vi "Parse.vi"(8 "error in (no error)":errorcluster, 11 "Multipart Parser in":refnum<class "Multipart Parser.lvclass">) -> (0 "error out":errorcluster, 1 "Stream":refnum<k5>, 3 "Request":refnum<class "Request.lvclass">)   [LabVIEW 2020, in "HTTP Utils.lvlib" / "Multipart Parser.lvclass"]
uses:
  Multipart Parser.lvclass
  Request/Request.lvclass
  Multipart Parser.lvclass/Multipart Parser.ctl
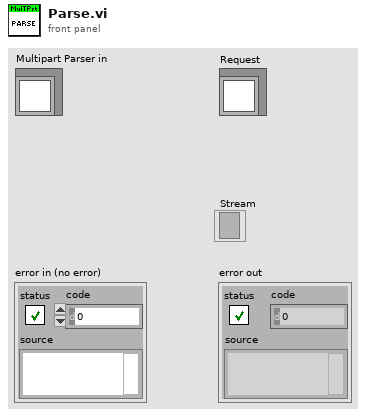
[diagram p1: front panel]
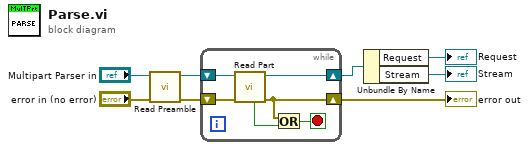
[diagram p0: block diagram]
diagram:
  n1 = call "Read Preamble.vi"("error in (no error)"="error in (no error)", "Multipart Parser in"="Multipart Parser in") -> ("error out"=w3:errorcluster, "Multipart Parser out"=w4:refnum<class "Multipart Parser.lvclass">)  [unwired: 8 in]
  n2 = while {
    shift-right: [w12] -> w2
    shift-left: w4 -> [w14]
    shift-right: [w9] -> w1
    shift-left: w3 -> [w13]
    stop <- w10 stop-if-true
    n3 = call "Read Part.vi"("error in (no error)"=w13, "Multipart Parser in"=w14) -> ("error out"=w9:errorcluster, "Multipart Parser out"=w12:refnum<class "Multipart Parser.lvclass">, "Last?"=w11:bool)  [unwired: 7 in]
    n4 = Or(x=w9, y=w11) -> (x .or. y?=w10:bool)
  }
  "error out" <- w1
  n5 = Unbundle By Name(w2) -> ("Request"=→"Request":refnum<class "Request.lvclass">, "Stream"=→"Stream":refnum<k5>)
